vi "Init.vi"(8 "error in (no error)":errorcluster, 10 "Initial Setting":variant, 11 "Hioki 9002 in":refnum<class "Hioki 9002.lvclass">) -> (0 "error out":errorcluster, 2 "Found?":bool=TRUE, 3 "Hioki 9002 out":refnum<class "Hioki 9002.lvclass">)   [LabVIEW 2025, in "Switch.lvlib" / "Hioki 9002.lvclass"]
uses:
  Hioki 9002.lvclass
  C:/Working copy/tss/Plugin/Engines/Switch/Switch Instrument/Switch Instrument.lvclass
  Users/Public/Documents/Sandia National Labs/TSS Plugin/Abstract Engine.lvlibp/Plugin/Abstract/Instrument configuration/Instrument configuration.lvclass
  Hioki 9002.lvclass/Hioki 9002.ctl
  Users/Public/Documents/Sandia National Labs/TSS Plugin/Abstract Engine.lvlibp/Plugin/Abstract/Instrument configuration/Read Instrument Setting.vi
  <instrlib>/HIOKI SW100X Series/Public/_Initialize/Initialize_USB.vi
  Users/Public/Documents/Sandia National Labs/TSS Plugin/CEF.lvlibp/serializable configuration/CEF_serializable configuration.lvclass
  <instrlib>/HIOKI SW100X Series/HIOKI SW100X Series.lvlib
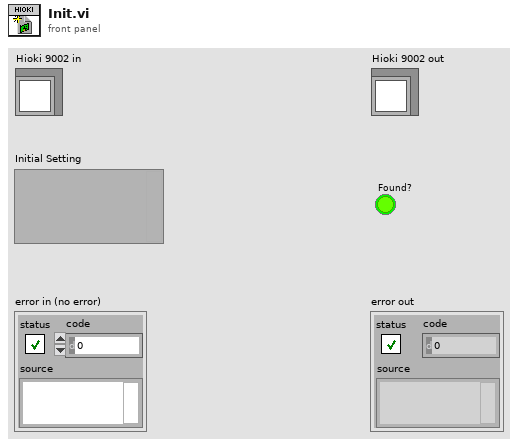
[diagram p1: front panel]
types:
  T1 = cluster{"Type":string, "Engine IP Address":string, "Engine Port":u32, "Address":string, "SW Alias":string, "Description":string, "Enabled":bool, "Model":string, "Serial Number":string, "Asset Number":string, "Calibration Date":string}
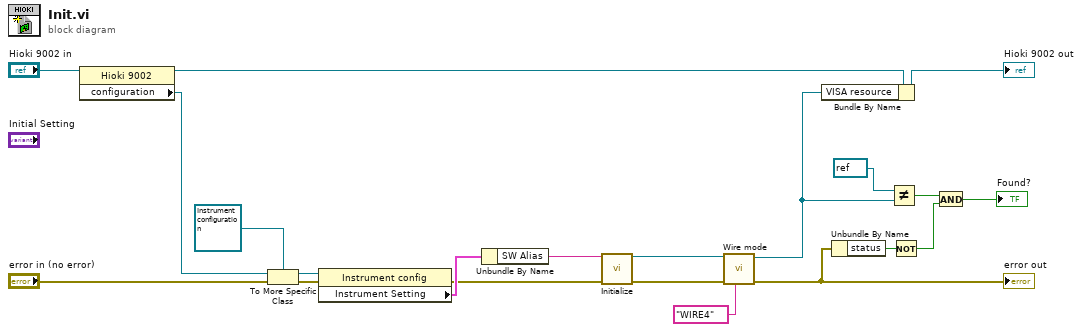
[diagram p0: block diagram]
diagram:
  n1 = property class="Hioki 9002"(reference="Hioki 9002 in") -> (reference out=w15:refnum<class "Hioki 9002.lvclass">, "configuration"=w17:refnum<class "CEF_serializable configuration.lvclass">)  [unwired: 1 in, 1 out]
  n2 = To More Specific Class(target class=refnum<class "Instrument configuration.lvclass"> refnum ("Abstract PlugIn.lvlibp:Instrument config"), reference=w17, error in="error in (no error)") -> (specific class reference=w20:refnum<class "Instrument configuration.lvclass">, error out=w21:errorcluster)
  n3 = property class="Instrument config"(reference=w20, error in=w21) -> (error out=w11:errorcluster, "Instrument Setting"=w16:T1)  [unwired: 1 out]
  n4 = Unbundle By Name(w16) -> ("SW Alias"=w10:string)
  n5 = call-poly <instrlib>:"Initialize.vi"("VISA resource name"=w10, "error in (no error)"=w11) -> ("VISA resource name out"=w9:refnum<visa-resource-name>, "error out"=w13:errorcluster)  [unwired: 11 in, 1 out]
  n6 = call <instrlib>:"Wire mode.vi"("Connection method"="WIRE4", "error in"=w13, "VISA resource name"=w9) -> ("error out"=w4:errorcluster, "VISA resource name out"=w7:refnum<visa-resource-name>)  [unwired: 6 in, 1 out]
  "error out" <- w4
  n7 = Bundle By Name(cluster=w15, "VISA resource"=w7) -> (→"Hioki 9002 out":refnum<class "Hioki 9002.lvclass">)
  n8 = Unbundle By Name(w4) -> ("status"=w5:bool)
  n9 = Not Equal?(x=refnum<visa-resource-name> refnum ("VISA resource"), y=w7) -> (x != y?=w3:bool)
  n10 = Not(x=w5) -> (.not. x?=w2:bool)
  n11 = And(x=w3, y=w2) -> (x .and. y?=→"Found?":bool)
